vi "EventLog.New(error).vi"(7 "Source (All)":T1, 8 "error in":errorcluster, 10 "ErrData":T2) -> (0 "error out":errorcluster)   [LabVIEW 2016]
uses:
  CitTemplate/citTemplate.errData.ctl
  EventLog.EventSource.ctl
  Translator/Translator.Message.ctl
  EventLog.EventGui.ctl
  EventLog.EventLevel.ctl
  EventLog.Buffer.Action.ctl
  EventLog.Event.ctl
  Global/ApplicationGlobal.vi
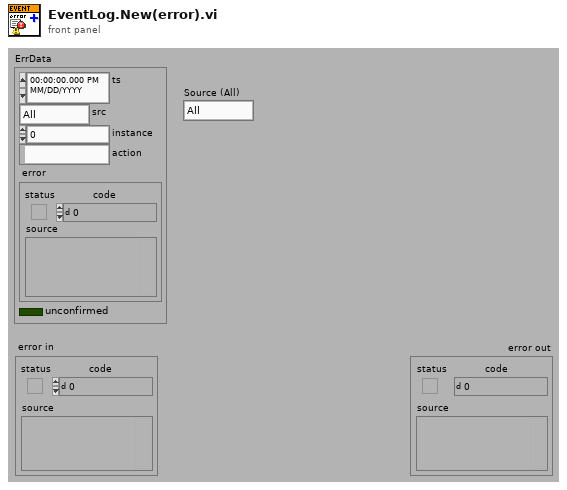
[diagram p1: front panel]
types:
  T1 = typedef "EventLog.EventSource.ctl" = enum16{"All", "Gui", "Cache", "PLC1", "PLC2", "PLC3", "DB", "DB01", "DB02", "DB03", "DB04", "DB05", "DB06", "DB07", "DB08", "DB09", "DB10", "DB11", "DB12", "DB13", "DB14", "DB15", "DB16"}
  T2 = typedef "citTemplate.errData.ctl" = cluster{"ts":timestamp, "src":T1, "instance":i32, "action":string, "error":errorcluster, "unconfirmed":bool}
  T3 = typedef "Translator.Message.ctl" = enum16{"-", "Event confirmed", "Log out", "Log in", "Shutdown", "Cancel", "Start", "Continue", "Stop", "On", "Off", "OK", "NOK", "NOK %s", "This", "Prev", "Home", "Work", "In progress...", "Missing", "Empty", "Hardware failure", "Initial", "Error %d >> %s", "Error %d >> %s >> %s", "Starting %s", "Quitting %s", "Configured", "Initializing", "Quitting", "Loading", "Running %s", "Stopped", "Summary", "Do you want to continue?", "Do you want to exit?", "Log out?", "System", "All", "IDLE", "Translating...%s", "Not found", "Alarm %s", "Run", "Skip", "Abort", "Repeat", "Please wait...", "Database disconnected", "Login to database successful", "Login to database failed: %d; %s", "Get process step data for %s", "Changeover off", "Changeover into %s", "Product %s | %s found in cache with status %d at previous station", "Product %s | %s found in database with status %d at previous station", "Product %s | %s not found in cache at previous station", "Product %s | %s not found in database at previous station", "Product %s | %s found in cache with status %d at this station (%d repetion)", "Product %s | %s found in database with status %d at this station (%d repetition)", "Product %s | %s not found in cache at this station", "Product %s | %s not found in database at this station", "Product %s | %s found in cache for component %s | %s", "Product %s | %s found in database for component %s | %s", "Product not found in cache for component %s | %s", "Product not found in database for component %s | %s", "Product %s | %s connected with component %s | %s (cache)", "Product %s | %s connected with component %s | %s (database)", "New data for %s | %s (cache)", "New data for %s | %s (database)", "File %s moved (cache)", "File %s deleted (cache)", "Msg %d >> %s", "PLC LifeBit Failure", "Reconnecting DB", "Reconnecting PLC", "Free disk space is below 1GB - contact technician", "Unable to check product status", "Product %s SN %s checked in DB", "Unable To check status from station %s"}
  T4 = typedef "EventLog.Event.ctl" = cluster{"ts":dbl, "lev":T5, "src":T1, "msg":T3, "arg":variant[]}
  T5 = typedef "EventLog.EventLevel.ctl" = enum8{"Debug", "Info", "Warning", "Error"}
  T6 = typedef "EventLog.Buffer.Action.ctl" = enum16{"init", "re-init", "clear", "set translator", "translate", "add", "get"}
  T7 = typedef "EventLog.EventGui.ctl" = cluster{"ts":dbl, "lev":T5, "src":T1, "msg":T3, "arg":variant[], "msg_str":string}
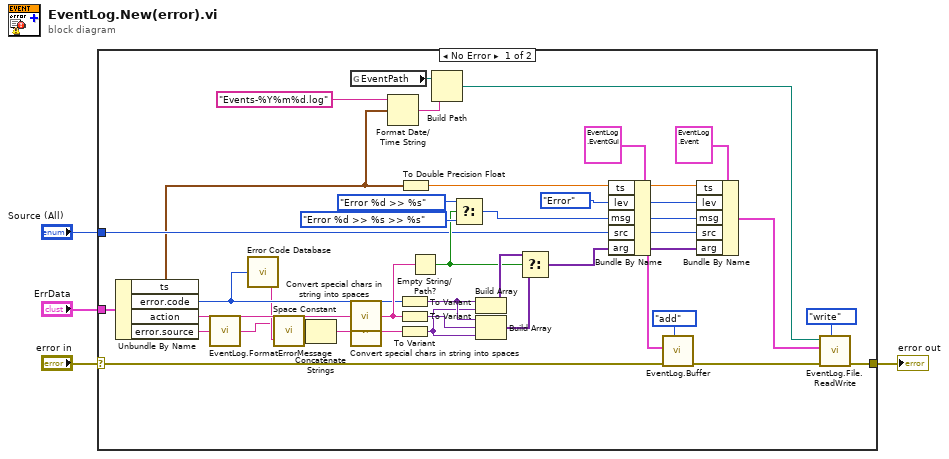
[diagram p0: block diagram]
diagram:
  n1 = case shown="No Error" "error in" {
    selector: "error in" -> [w14 w42]
    tunnel: [w38 w42] -> w4
    tunnel: "ErrData" -> [w30 _]
    tunnel: "Source (All)" -> [w17 _]
    frame No Error {
      w15 = EventLog.EventLevel."Error" ("lev")
      n2 = Unbundle By Name(w30) -> ("ts"=w12:timestamp, "error.code"=w11:i32, "action"=w29:string, "error.source"=w7:string)
      n3 = call "EventLog.FormatErrorMessage.vi"("Error string in"=w7) -> ("Error string out"=w6:string)
      n4 = call <vilib>:"Error Code Database.vi"("Error Code"=w11) -> ("Error Text"=w8:string)
      n5 = call <vilib>:"Space Constant.vi"() -> ("String"=w9:string)
      n6 = Concatenate Strings(w6, w9, w8) -> (w10:string)
      n7 = global read "ApplicationGlobal.vi" "EventPath"() -> (w33:path)
      n8 = call "Convert special chars in string into spaces.vi"("string with special characters"=w29) -> ("string with spaces"=w27:string)  [unwired: 2 in]
      n9 = call "Convert special chars in string into spaces.vi"("string with special characters"=w10) -> ("string with spaces"=w28:string)  [unwired: 2 in]
      n10 = Format Date/Time String(time format string (%c)="Events-%Y%m%d.log", seconds (now)=w12) -> (date/time string=w32:string)  [unwired: 1 in]
      n11 = To Variant(anything=w11) -> (Variant=w25:variant)
      n12 = To Variant(anything=w27) -> (Variant=w24:variant)
      n13 = To Variant(anything=w28) -> (Variant=w23:variant)
      n14 = To Double Precision Float(number=w12) -> (double precision float=w36:dbl)
      n15 = Empty String/Path?(string/path=w27) -> (empty?=w18:bool)
      n16 = Build Path(base path=w33, name or relative path=w32) -> (appended path=w31:path)
      n17 = Select(t=Translator.Message."Error %d >> %s" ("msg"), s=w18, f=Translator.Message."Error %d >> %s >> %s" ("msg")) -> (s? t:f=w5:T3)
      n18 = Build Array(w25, w23) -> (w26:variant[])
      n19 = Build Array(w25, w24, w23) -> (w22:variant[])
      n20 = Select(t=w26, s=w18, f=w22) -> (s? t:f=w21:variant[])
      n21 = Bundle By Name(cluster=T7 {"ts"=0.0, "lev"=enum."Debug", "src"=enum."All", "msg"=enum."Log out", "arg"=[], "msg_str"=""} ("Event in"), "ts"=w36, "lev"=w15, "msg"=w5, "src"=w17, "arg"=w21) -> (w16:T7)
      n22 = call "EventLog.Buffer.vi"("action (get)"=EventLog.Buffer.Action."add" ("action (read)"), "error in"=w14, "Event in"=w16) -> ("error out"=w13:errorcluster)  [unwired: 5 in, 3 out]
      n23 = Bundle By Name(cluster=T4 {"ts"=0.0, "lev"=enum."Debug", "src"=enum."All", "msg"=enum."Log out", "arg"=[]} ("event in"), "ts"=w36, "lev"=w15, "msg"=w5, "src"=w17, "arg"=w21) -> (w35:T4)
      n24 = call "EventLog.File.ReadWrite.vi"("action (read)"=enum16{"read", "write"}."write", "error in"=w13, "event in"=w35, "file"=w31) -> ("error out"=w38:errorcluster)  [unwired: 3 in, 4 out]
    }
    frame Error {
    }
  }
  "error out" <- w4
